vi "Tactile Illusions Control System.vi"() -> ()   [LabVIEW 2020]
uses:
  <vilib>/Waveform/WDTOps.llb/WDT Append Waveforms DBL.vi
  <vilib>/Waveform/WDTFileIO.llb/Export Waveforms To Spreadsheet File (1D).vi
panel:
  in  "Cell Opened":bool
  in  "VISA resource name in 4":refnum<visa-resource-name>
  in  "VISA resource name in 3":refnum<visa-resource-name>
  in  "Stop Acquisition":bool
  in  "Enable save":bool
  out "Voltage":waveform(dbl)(graph)
  out "Temperature":waveform(dbl)(graph)
  out "Voltage and Temperature":waveform(dbl)[](graph)
  out "size(10) 2":i32
  out "size(x10) 2":i32
  out "size(x10)":i32
  out "size(10)":i32
  out "Current Control":dbl
  out "size(10) 3":i32
  out "Calibrated Temperature":dbl
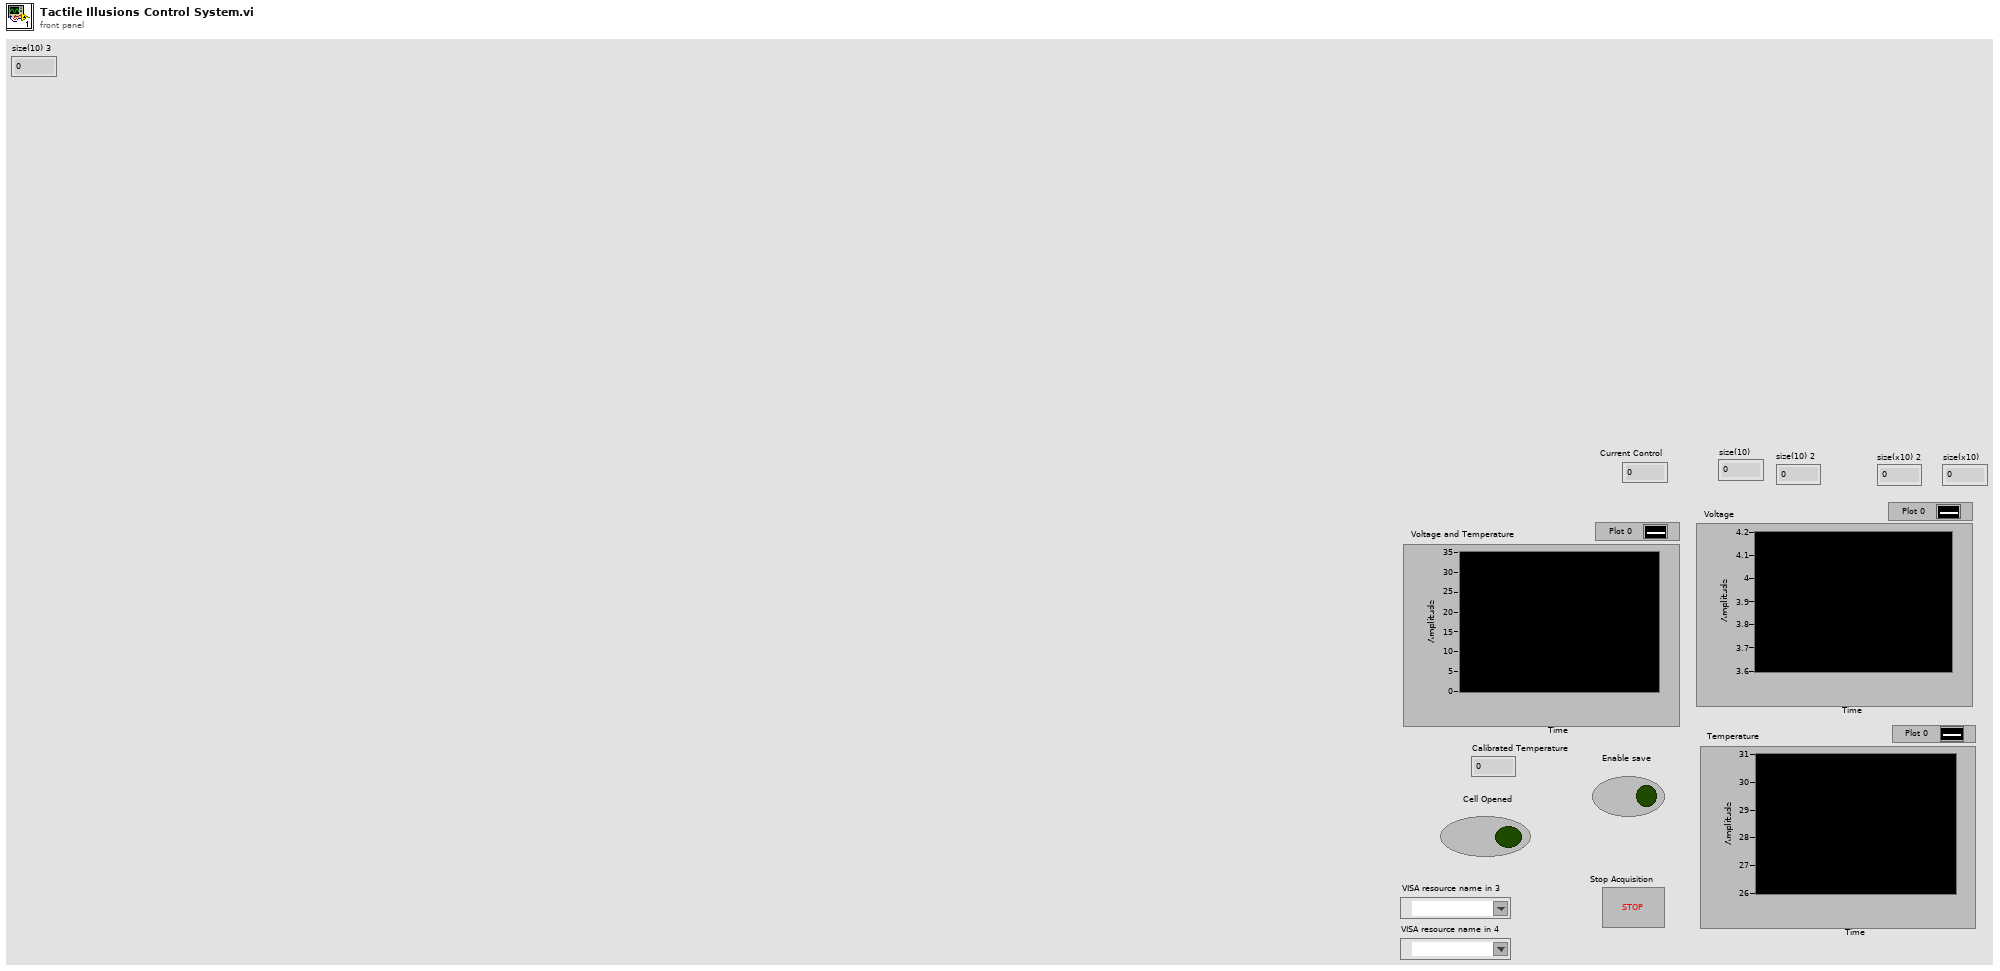
[diagram p1: front panel]
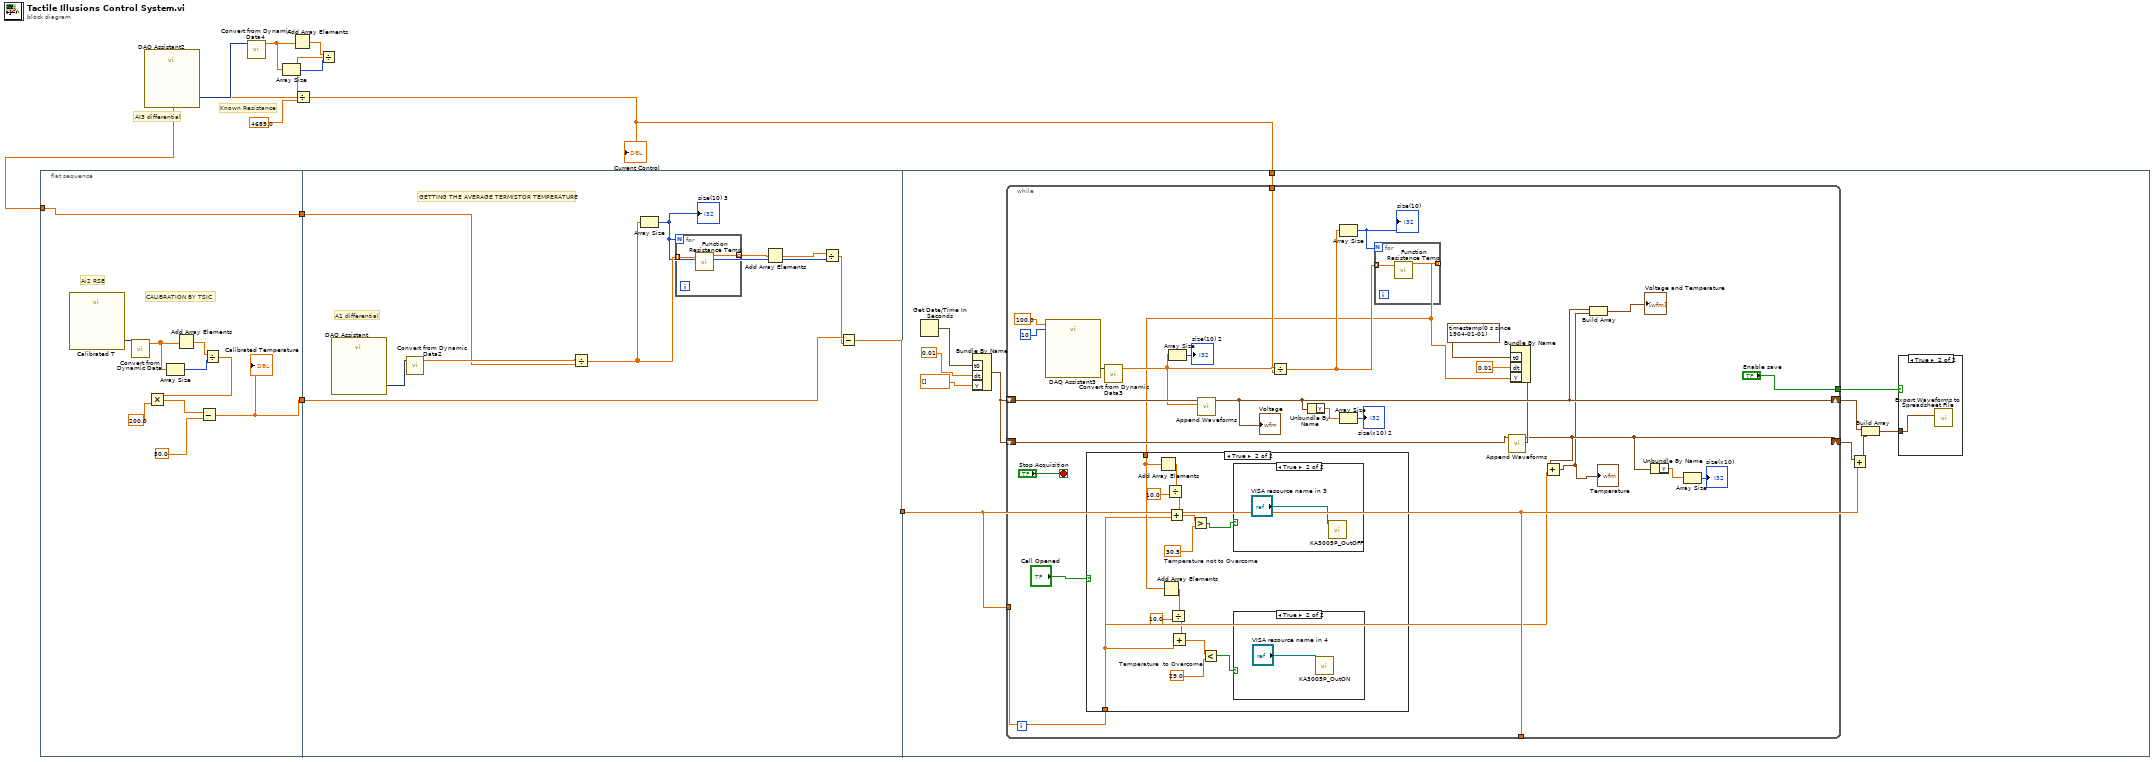
[diagram p0: block diagram]
diagram:
  # "AI3 differential"
  # "Known Resistance"
  n1 = flat-sequence {
    tunnel: [w13] -> w10
    tunnel: w2 -> [w11]
    tunnel: [w11] -> w9
    tunnel: w10 -> [w25]
    tunnel: w9 -> [w22]
    tunnel: [w21] -> w1
    tunnel: w2 -> [w36]
    tunnel: w1 -> [w33]
    frame #0 {
      # "Ai2 RSE"
      # "CALIBRATION BY TSIC"
      n2 = call "Calibrated T"() -> ("data"=w12:dynamicdata)  [unwired: 17 in, 2 out]
      n3 = call "Convert from Dynamic Data"("Dynamic Data Type"=w12) -> ("Array"=w17:dbl[])  [unwired: 3 in]
      n4 = Array Size(array=w17) -> (size(s)=w15:i32)
      n5 = Add Array Elements(numeric array=w17) -> (sum=w16:dbl)
      n6 = Divide(x=w16, y=w15) -> (x/y=w14:dbl)
      n7 = Multiply(x=w14, y=200.0) -> (x*y=w19:dbl)
      n8 = Subtract(x=w19, y=50.0) -> (x-y=w13:dbl)
      "Calibrated Temperature" <- w13
    }
    frame #1 {
      # "A1 differential"
      # "GETTING THE AVERAGE TERMISTOR TEMPERATURE"
      n9 = call "DAQ Assistant"() -> ("data"=w23:dynamicdata)  [unwired: 17 in, 2 out]
      n10 = call "Convert from Dynamic Data2"("Dynamic Data Type"=w23) -> ("Array"=w29:dbl[])  [unwired: 3 in]
      n11 = Divide(x=w29, y=w22) -> (x/y=w30:dbl[])
      n12 = Array Size(array=w30) -> (size(s)=w26:i32)
      "size(10) 3" <- w26
      n13 = for {
        N: w26 -> [_]
        tunnel: w30 -> [w32] mode=indexing
        tunnel: [w31] -> w28 mode=indexing
        n14 = call "Function Resistance Temp.vi"("Resistance"=w32) -> ("y"=w31:dbl)  [unwired: 10 in]
      }
      n15 = Add Array Elements(numeric array=w28) -> (sum=w27:dbl)
      n16 = Divide(x=w27, y=w26) -> (x/y=w24:dbl)
      n17 = Subtract(x=w25, y=w24) -> (x-y=w21:dbl)
    }
    frame #2 {
      n18 = Get Date/Time In Seconds() -> (seconds since 1Jan1904=w39:timestamp)
      n19 = Bundle By Name("t0"=w39, "dt"=0.01, "Y"=dbl[] []) -> (w41:waveform(dbl))  [unwired: 1 in]
      n20 = while {
        shift-right: [w57] -> w42
        shift-left: w41 -> [w68]
        tunnel: ["Enable save"] -> w40
        shift-right: [w48] -> w35
        shift-left: w41 -> [w49]
        tunnel: w36 -> [w51]
        tunnel: w33 -> [_]
        tunnel: w33 -> [w45]
        stop <- "Stop Acquisition" stop-if-true
        n21 = call "DAQ Assistant3"("rate"=100.0, "number of samples"=10) -> ("data"=w67:dynamicdata)  [unwired: 14 in, 3 out]
        n22 = call "Convert from Dynamic Data3"("Dynamic Data Type"=w67) -> ("Array"=w52:dbl[])  [unwired: 3 in]
        n23 = Array Size(array=w52) -> (size(s)=→"size(10) 2":i32)
        n24 = call-poly <vilib>:"Append Waveforms.vi"("waveform B"=w52, "waveform A"=w68) -> ("waveform out"=w57:waveform(dbl))  [unwired: 8 in, 1 out]
        "Voltage" <- w57
        n25 = Divide(x=w52, y=w51) -> (x/y=w63:dbl[])
        n26 = Unbundle By Name(w57) -> ("Y"=w56:dbl[])
        n27 = Array Size(array=w63) -> (size(s)=w62:i32)
        "size(10)" <- w62
        n28 = Array Size(array=w56) -> (size(s)=→"size(x10) 2":i32)
        n29 = for {
          N: w62 -> [_]
          tunnel: w63 -> [w87] mode=indexing
          tunnel: [w86] -> w46 mode=indexing
          n30 = call "Function Resistance Temp.vi"("Resistance"=w87) -> ("y"=w86:dbl)  [unwired: 10 in]
        }
        n31 = case shown="True" "Cell Opened" {
          tunnel: w46 -> [_ w71]
          tunnel: w45 -> [_ w70]
          frame False {
          }
          frame True {
            w74 = 29.0  # Temperature  to Overcome
            w79 = 30.5  # Temperature not to Overcome
            n32 = Add Array Elements(numeric array=w71) -> (sum=w82:dbl)
            n33 = Add Array Elements(numeric array=w71) -> (sum=w76:dbl)
            n34 = Divide(x=w82, y=10.0) -> (x/y=w81:dbl)
            n35 = Add(x=w81, y=w70) -> (x+y=w78:dbl)
            n36 = Divide(x=w76, y=10.0) -> (x/y=w75:dbl)
            n37 = Add(x=w75, y=w70) -> (x+y=w73:dbl)
            n38 = Greater?(x=w78, y=w79) -> (0:w80:bool)
            n39 = Less?(x=w73, y=w74) -> (x < y?=w72:bool)
            n40 = case shown="True" w80 {
              frame False {
              }
              frame True {
                n41 = call <vilib>:"KA3005P_OutOFF.vi"("VISA resource name in"="VISA resource name in 3") -> ()  [unwired: 9 in, 2 out]
              }
            }
            n42 = case shown="True" w72 {
              frame False {
              }
              frame True {
                n43 = call <vilib>:"KA3005P_OutON.vi"("VISA resource name in"="VISA resource name in 4") -> ()  [unwired: 9 in, 2 out]
              }
            }
          }
        }
        n44 = Bundle By Name("t0"=timestamp(0 s since 1904-01-01), "dt"=0.01, "Y"=w46) -> (w50:waveform(dbl))  [unwired: 1 in]
        n45 = call-poly <vilib>:"Append Waveforms.vi"("waveform B"=w50, "waveform A"=w49) -> ("waveform out"=w48:waveform(dbl))  [unwired: 8 in, 1 out]
        n46 = Add(x=w48, y=w45) -> (x+y=w47:waveform(dbl))
        "Temperature" <- w47
        n47 = Build Array(w57, w47) -> (→"Voltage and Temperature":waveform(dbl)[])
        n48 = Unbundle By Name(w48) -> ("Y"=w53:dbl[])
        n49 = Array Size(array=w53) -> (size(s)=→"size(x10)":i32)
      }
      n50 = Add(x=w35, y=w33) -> (x+y=w34:waveform(dbl))
      n51 = Build Array(w42, w34) -> (w43:waveform(dbl)[])
      n52 = case shown="True" w40 {
        tunnel: w43 -> [_ w88]
        frame False {
        }
        frame True {
          n53 = call-poly <vilib>:"Export Waveforms to Spreadsheet File.vi"("waveforms"=w88) -> ()  [unwired: 9 in, 2 out]
        }
      }
    }
  }
  n54 = call "DAQ Assistant2"() -> ("data"=w3:dynamicdata)  [unwired: 17 in, 2 out]
  n55 = call "Convert from Dynamic Data4"("Dynamic Data Type"=w3) -> ("Array"=w7:dbl[])  [unwired: 3 in]
  n56 = Array Size(array=w7) -> (size(s)=w5:i32)
  n57 = Add Array Elements(numeric array=w7) -> (sum=w6:dbl)
  n58 = Divide(x=w6, y=w5) -> (x/y=w4:dbl)
  n59 = Divide(x=w4, y=4689.0) -> (x/y=w2:dbl)
  "Current Control" <- w2
